vi "Find and parse list line.vi"(8 "Error In":errorcluster, 10 "Property":string, 11 "String":string) -> (0 "Error Out":errorcluster, 3 "List":string[](array[string]))   [LabVIEW 2015]
uses:
  <vilib>/regexp/Match Regular Expression.xnode
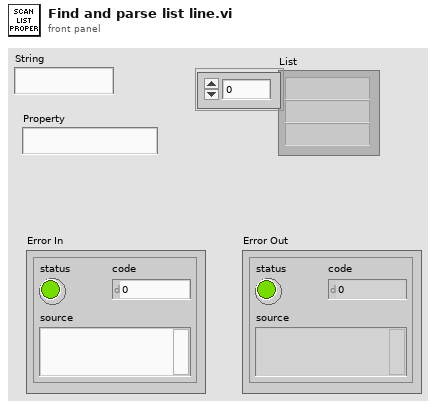
[diagram p1: front panel]
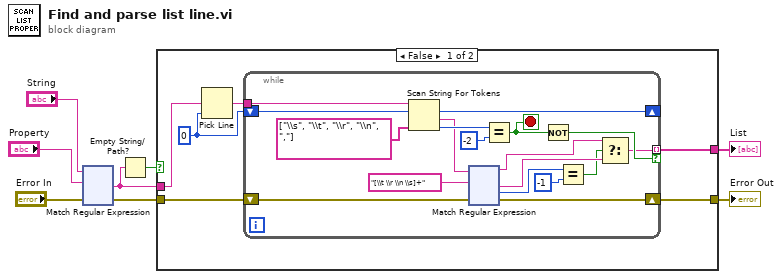
[diagram p0: block diagram]
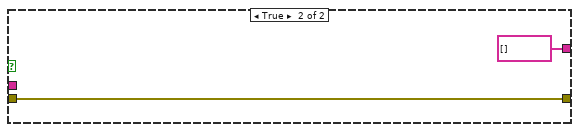
[diagram p2: hidden frame]
diagram:
  n1 = xnode "Match Regular Expression"("input string"="String", "regular expression"="Property", "error in"="Error In") -> ("after match"=w7:string, "error out"=w2:errorcluster)  [unwired: 3 in, 3 out]
  n2 = Empty String/Path?(string/path=w7) -> (empty?=w6:bool)
  n3 = case shown="False" w6 {
    tunnel: w7 -> [w14 _]
    tunnel: [w12 string[] []] -> w8
    tunnel: w2 -> [w11 w144]
    tunnel: [w10 w144] -> w1
    frame False {
      w9 = 0 ("line index")
      n4 = Pick Line(multi-line string=w14, line index=w9) -> (output string=w13:string)  [unwired: 1 in]
      n5 = while {
        tunnel: w13 -> [w28]
        shift-right: [w32] -> _
        shift-left: w9 -> [w27]
        tunnel: [w20] -> w12 mode=indexing if=w26
        shift-right: [w15] -> w10
        shift-left: w11 -> [w16]
        stop <- w29 stop-if-true
        n6 = Scan String For Tokens(6:string[] ["\\s", "\\t", "\\r", "\\n", ","] ("delimiters (\\s,\\t,\\r,\\n)"), 8:w27, 9:w28) -> (0:w31:i32, 1:w24:string, 2:w32:i32)  [unwired: 3 in, 1 out]
        n7 = xnode "Match Regular Expression"("input string"=w24, "regular expression"="[\\t \\r \\n \\s]+", "error in"=w16) -> ("before match"=w19:string, "after match"=w18:string, "offset past match"=w22:i32, "error out"=w15:errorcluster)  [unwired: 3 in, 1 out]
        n8 = Equal?(x=w31, y=-2) -> (x = y?=w29:bool)
        n9 = Not(x=w29) -> (.not. x?=w26:bool)
        n10 = Equal?(x=w22, y=-1) -> (x = y?=w17:bool)
        n11 = Select(t=w19, s=w17, f=w18) -> (s? t:f=w20:string)
      }
    }
    frame True {
    }
  }
  "List" <- w8
  "Error Out" <- w1
